vi "Check Packet.vi"(1 "Serial":u8[](array[numeric])) -> (0 "Packet?":bool)   [LabVIEW 2011]
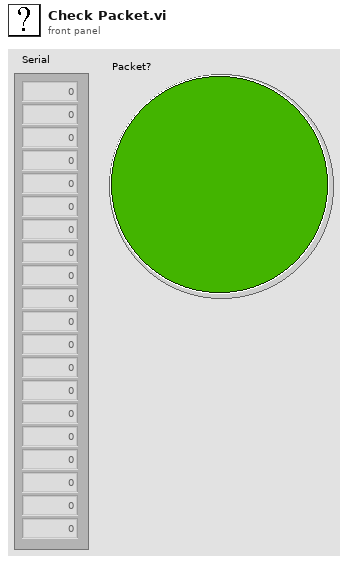
[diagram p1: front panel]
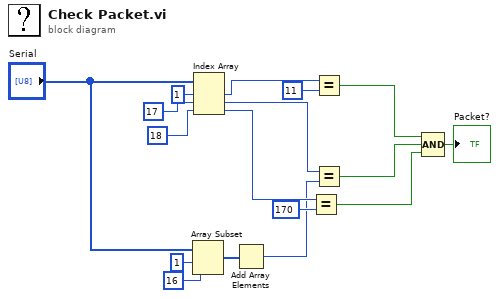
[diagram p0: block diagram]
diagram:
  n1 = Array Subset(array="Serial", index=1 ("인덱스"), length=16 ("길이")) -> (w8:u8[])
  n2 = Index Array(array="Serial", index #1=1 ("인덱스"), index #2=17 ("인덱스"), index #3=18 ("인덱스")) -> (element #1=w6:u8, element #2=w12:u8, element #3=w14:u8)
  n3 = Add Array Elements(numeric array=w8) -> (sum=w7:u8)
  n4 = Equal?(x=w14, y=u8 170) -> (x = y?=w2:bool)
  n5 = Equal?(x=w6, y=u8 11) -> (x = y?=w4:bool)
  n6 = Equal?(x=w12, y=w7) -> (x = y?=w3:bool)
  n7 = Compound Arithmetic op=AND(w4, w3, w2) -> (→"Packet?":bool)
